vi "Cleanup.vi"(8 "error in (no error)":errorcluster, 11 "Class In":refnum<class "Time Step.lvclass">) -> (0 "error out":errorcluster, 3 "Class Out":refnum<class "Time Step.lvclass">)   [LabVIEW 2018, in "Temp Recipe.lvlib" / "Time Step.lvclass"]
uses:
  Time Step.lvclass
  Time Step.lvclass/Time Step.ctl
  Ref Data.ctl
  Recipe Step/Recipe Step.lvclass
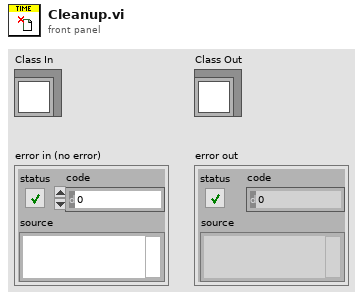
[diagram p1: front panel]
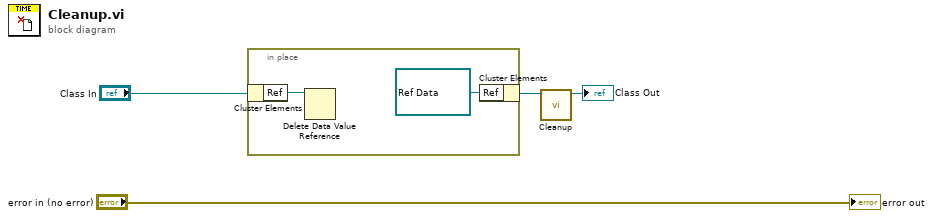
[diagram p0: block diagram]
diagram:
  n1 = in-place {
    n2 = in-place-cluster #1("Class In") -> ("Ref"=w6:refnum<data-value>)
    n3 = Delete Data Value Reference(data value reference=w6) -> ()  [unwired: 1 in, 2 out]
    n4 = in-place-cluster #1("Ref"=refnum<data-value> refnum) -> (w2:refnum<class "Time Step.lvclass">)
  }
  n5 = call-parent "Cleanup.vi"("Panel in"=w2) -> ("Panel out"=→"Class Out":refnum<class "Time Step.lvclass">)  [unwired: 9 in, 1 out]
  "error out" <- "error in (no error)"
